vi "CheckReference.vi"(0 "reference":refnum<class "VdTcpIP.lvclass">, 5 "error in (no error)":errorcluster) -> (14 "reference out":refnum<class "VdTcpIP.lvclass">, 15 "Not a Refnum":bool, 19 "error out":errorcluster)   [LabVIEW 2020, in "VdTcpIP.lvclass"]
doc: "Reads a message"
uses:
  VdTcpIP.lvclass
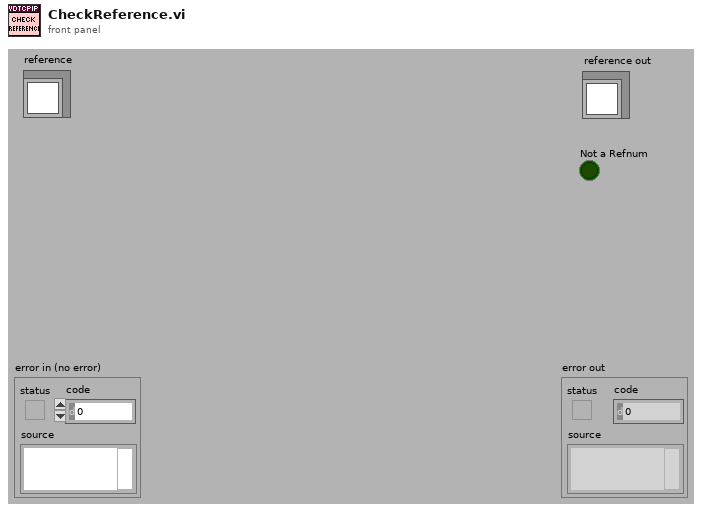
[diagram p1: front panel]
types:
  T1 = typedef "VdTcpIP.lvclass/ObjectAttributes.ctl" = cluster{"IP-Address":string, "Port":u16, "Connection":refnum<k5>, "Listener":refnum<k5>, "ListenerConnection":refnum<k5>, "Listner":bool, "ListnerProcessRunning":bool, "InConnections":refnum<k5>[], "InConnectionsIP":string[], "InConnectionAdded":refnum<notifier>, "RunVIOnNewConnection":variant, "DataToNewConnectionVI":cluster{"ControlName":string, "ControlValue":variant}[], "WebServicesURL_Location(http://...)":string, "WebServicesPostWebPage(*.asmx)":string, "Semaphore":T2, "AutoReConnectTimes":i32, "AutoReConnectInterval(ms)":i32, "ConnectionTimeout":i32}
  T2 = typedef "Semaphore RefNum" = refnum<k1>
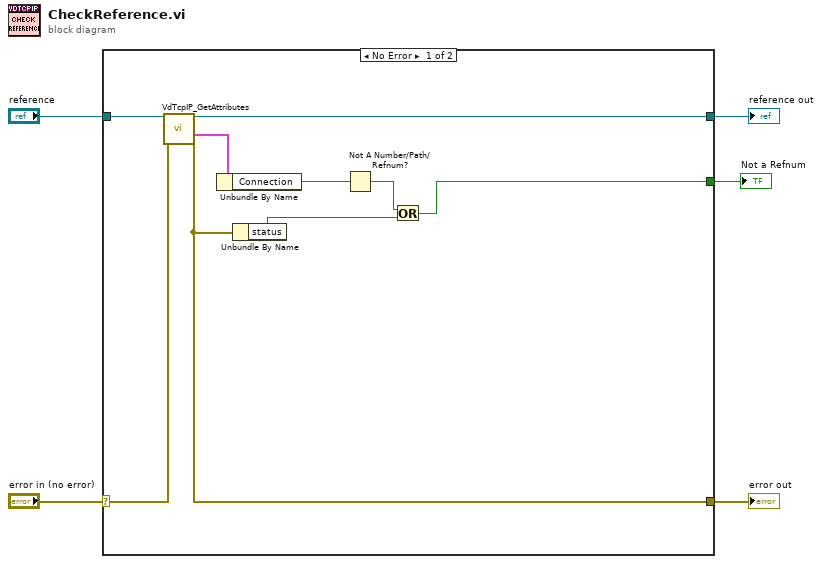
[diagram p0: block diagram]
diagram:
  n1 = case shown="No Error" "error in (no error)" {
    selector: "error in (no error)" -> [w14 w15]
    tunnel: "reference" -> [w13 w16]
    tunnel: [w10 w15] -> w3
    tunnel: [w12 w16] -> w2
    tunnel: [w7 _] -> w1
    frame No Error {
      n2 = call "VdTcpIP_GetAttributes.vi"("reference in"=w13, "error in (no error)"=w14) -> ("reference out"=w12:refnum<class "VdTcpIP.lvclass">, "Data"=w6:T1, "error out"=w10:errorcluster)  [unwired: 1 in, 14 out]
      n3 = Unbundle By Name(w6) -> ("Connection"=w11:refnum<k5>)
      n4 = Unbundle By Name(w10) -> ("status"=w9:bool)
      n5 = Not A Number/Path/Refnum?(number/path/refnum=w11) -> (NaN/Path/Refnum?=w8:bool)
      n6 = Or(x=w8, y=w9) -> (x .or. y?=w7:bool)
    }
    frame Error {
    }
  }
  "reference out" <- w2
  "error out" <- w3
  "Not a Refnum" <- w1
